vi "LaguerreGaussianBeam.vi"(0 "beam parameters":T1={"amplitudeMatrix"=[], "SLM width (m)"=0.01498, "SLM height (m)"=0.01092, "wavelength (m)"=6.33e-07, "Resolution x"=1920, "Resolution y"=1080} caption="Beam Parameters, dependant on SLM and LASER" {"Resolution x" format="%#.0f"; "SLM width (m)" format="%_6f"; "SLM height (m)" format="%#_6f"}, 1 "x centre":dbl, 2 "l":i16, 3 "p":i16 min=0 step=1, 4 "beam waist w0 (in m; default 1E-4 = 0.1mm)":dbl=0.0001 format="%.2p", 5 "Phase rotation":dbl min=-6.2832 max=6.28318530718 step=0.01570796326, 6 "y centre":dbl, 7 "Correction beam waist wc \n(in m; default 1 meter)":dbl=1.0 format="%.2p") -> (8 "Laguerre-Gaussian beam":T1={"amplitudeMatrix"=[], "SLM width (m)"=0.01498, "SLM height (m)"=0.01092, "wavelength (m)"=6.33e-07, "Resolution x"=1920, "Resolution y"=1080} caption="Beam Parameters, dependant on SLM and LASER" {"Resolution x" format="%#.0f"; "SLM width (m)" format="%_6f"; "SLM height (m)" format="%#_6f"})   [LabVIEW 2024]
uses:
  typeDefs/BPandSLM.ctl
panel:
  out "min value":dbl
  out "max value":dbl
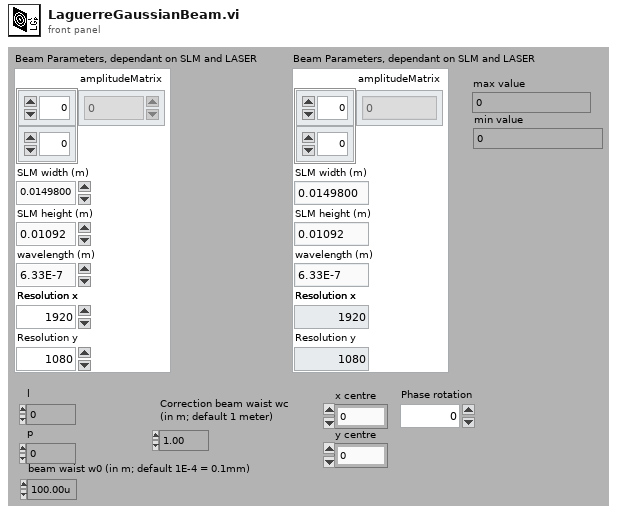
[diagram p1: front panel]
types:
  T1 = typedef "BPandSLM.ctl" = cluster{"amplitudeMatrix":csg[][], "SLM width (m)":dbl, "SLM height (m)":dbl, "wavelength (m)":dbl, "Resolution x":u32, "Resolution y":u32}
  T2 = cluster{"x values":dbl[], "laguerre polynomial values":dbl[]}
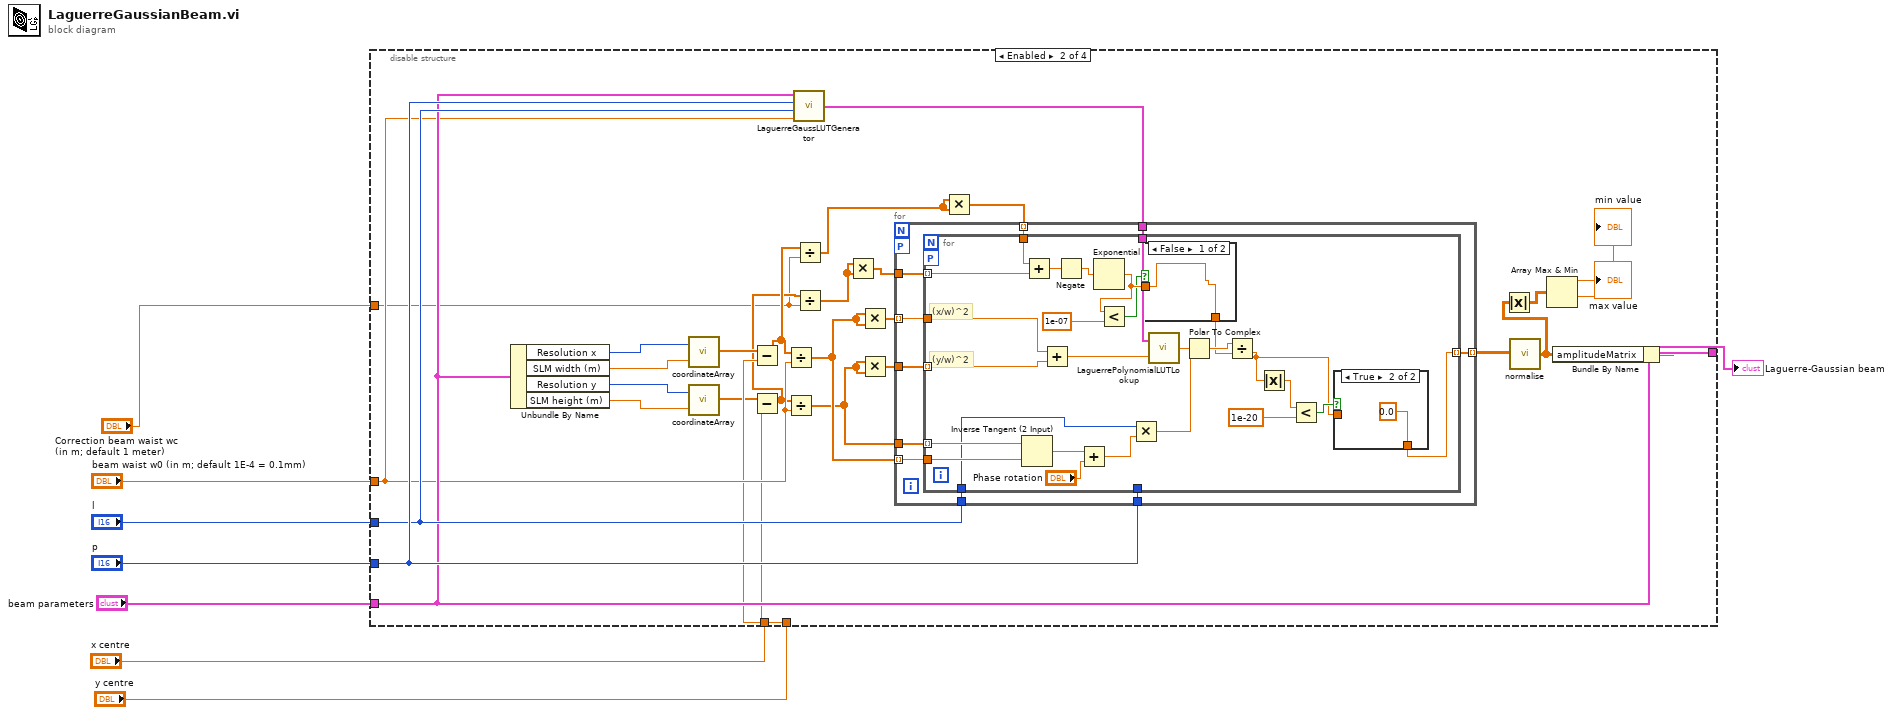
[diagram p0: block diagram]
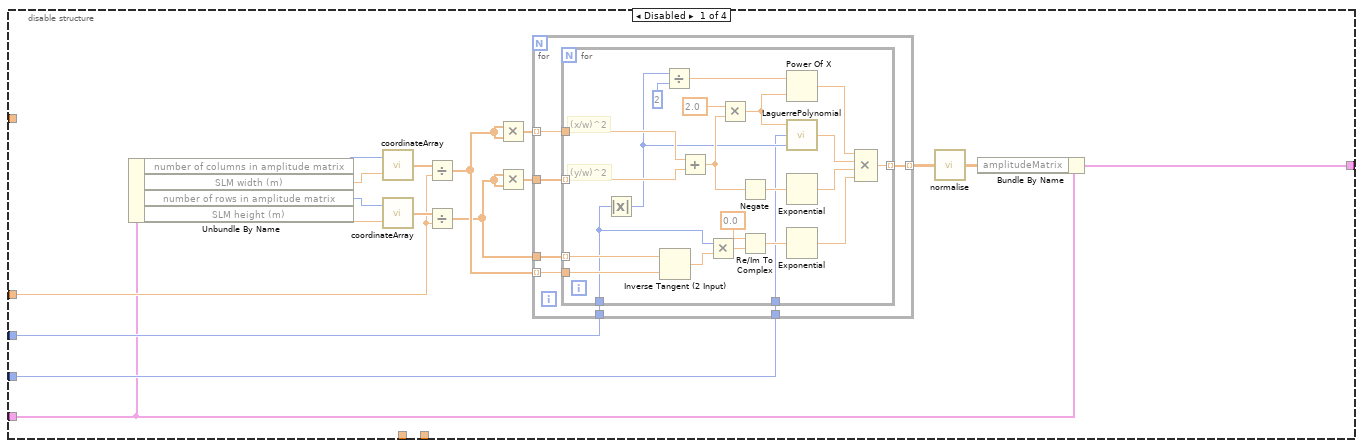
[diagram p2: hidden frame]
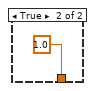
[diagram p4: hidden frame]
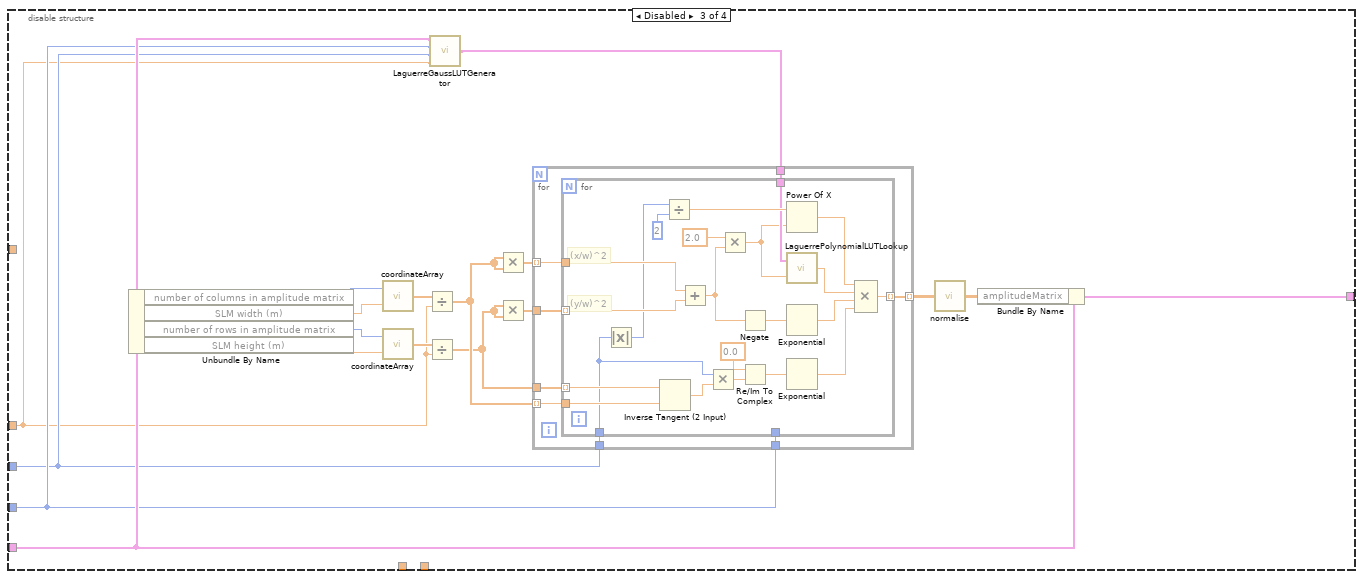
[diagram p5: hidden frame]
diagram:
  n1 = disable-structure shown="Enabled" {
    disable-tunnel: [w25 w84 w142 _] -> w2
    disable-tunnel: "p" -> [w12 w77 w127 _]
    disable-tunnel: "l" -> [w11 w76 w126 _]
    disable-tunnel: "beam waist w0 (in m; default 1E-4 = 0.1mm)" -> [w10 w74 w125 _]
    disable-tunnel: "beam parameters" -> [w9 w75 w128 _]
    disable-tunnel: "x centre" -> [_ w71 _ _]
    disable-tunnel: "y centre" -> [_ w72 _ _]
    disable-tunnel: "Correction beam waist wc \n(in m; default 1 meter)" -> [_ w64 _ _]
    frame Disabled {
      n2 = Unbundle By Name(w9) -> ("number of columns in amplitude matrix"=w24:i32, "SLM width (m)"=w14:dbl, "number of rows in amplitude matrix"=w23:i32, "SLM height (m)"=w13:dbl)
      n3 = call "coordinateArray.vi"("width of represented x (or y) range (in m; default 1E-3=1mm)"=w14, "array size (default 64)"=w24) -> ("x array"=w22:sgl[])
      n4 = call "coordinateArray.vi"("width of represented x (or y) range (in m; default 1E-3=1mm)"=w13, "array size (default 64)"=w23) -> ("x array"=w21:sgl[])
      n5 = Divide(x=w22, y=w10) -> (x/y=w18:dbl[])
      n6 = Divide(x=w21, y=w10) -> (x/y=w17:dbl[])
      n7 = Multiply(x=w18, y=w18) -> (x*y=w20:dbl[])
      n8 = Multiply(x=w17, y=w17) -> (x*y=w19:dbl[])
      n9 = for {
        tunnel: [w32] -> w16 mode=indexing
        tunnel: w20 -> [w31] mode=indexing
        tunnel: w19 -> [w30]
        tunnel: w18 -> [w29] mode=indexing
        tunnel: w17 -> [w28]
        tunnel: w11 -> [w27]
        tunnel: w12 -> [w26]
        n10 = for {
          tunnel: [w53] -> w32 mode=indexing
          tunnel: w31 -> [w52]
          tunnel: w30 -> [w51] mode=indexing
          tunnel: w29 -> [w41]
          tunnel: w28 -> [w40] mode=indexing
          tunnel: w27 -> [w37]
          tunnel: w26 -> [w33]
          # "(y/w)^2"
          # "(x/w)^2"
          n11 = Absolute Value(x=w37) -> (abs(x)=w34:i16)
          n12 = Inverse Tangent (2 Input)(1:w41, 2:w40) -> (0:w44:dbl)
          n13 = Divide(x=w34, y=i16 2) -> (x/y=w38:dbl)
          n14 = Add(x=w52, y=w51) -> (x+y=w48:dbl)
          n15 = Multiply(x=w37, y=w44) -> (x*y=w45:dbl)
          n16 = Multiply(x=2.0, y=w48) -> (x*y=w35:dbl)
          n17 = Negate(x=w48) -> (-x=w54:dbl)
          n18 = Re/Im To Complex(1:w45, 2:0.0 ("x")) -> (0:w46:cdb)
          n19 = Power Of X(1:w35, 2:w38) -> (0:w49:dbl)
          n20 = call "LaguerrePolynomial.vi"("a"=w34, "n"=w33, "x"=w35) -> ("associated Laguerre polynomial (n,a,x)"=w36:dbl)
          n21 = Exponential(1:w54) -> (0:w47:dbl)
          n22 = Exponential(1:w46) -> (0:w42:cdb)
          n23 = Compound Arithmetic op=MULTIPLY(w49, w36, w47, w42) -> (w53:cdb)
        }
      }
      n24 = call "normalise.vi"("amplitude matrix"=w16) -> ("normalised amplitude matrix"=w15:cdb[][])
      n25 = Bundle By Name(cluster=w9, "amplitudeMatrix"=w15) -> (w25:T1)
    }
    frame Enabled {
      n26 = Unbundle By Name(w75) -> ("Resolution x"=w83:u32, "SLM width (m)"=w79:dbl, "Resolution y"=w82:u32, "SLM height (m)"=w78:dbl)
      n27 = call "coordinateArray.vi"("width of represented x (or y) range (in m; default 1E-3=1mm)"=w79, "array size (default 64)"=w83) -> ("x array"=w70:sgl[])
      n28 = call "coordinateArray.vi"("width of represented x (or y) range (in m; default 1E-3=1mm)"=w78, "array size (default 64)"=w82) -> ("x array"=w67:sgl[])
      n29 = Subtract(x=w70, y=w71) -> (x-y=w66:dbl[])
      n30 = Subtract(x=w67, y=w72) -> (x-y=w65:dbl[])
      n31 = Divide(x=w66, y=w74) -> (x/y=w69:dbl[])
      n32 = Divide(x=w65, y=w74) -> (x/y=w68:dbl[])
      n33 = call "LaguerreGaussLUTGenerator.vi"("beam waist w0 (in m; default 1E-4 = 0.1mm)"=w74, "l"=w76, "p"=w77, "beam parameters"=w75) -> ("Look-up Table"=w73:T2)
      n34 = Divide(x=w66, y=w64) -> (x/y=w62:dbl[])
      n35 = Divide(x=w65, y=w64) -> (x/y=w63:dbl[])
      n36 = Multiply(x=w63, y=w63) -> (x*y=w60:dbl[])
      n37 = Multiply(x=w69, y=w69) -> (x*y=w81:dbl[])
      n38 = Multiply(x=w68, y=w68) -> (x*y=w80:dbl[])
      n39 = Multiply(x=w62, y=w62) -> (x*y=w61:dbl[])
      n40 = for {
        tunnel: [w94] -> w55 mode=indexing
        tunnel: w81 -> [w93] mode=indexing
        tunnel: w80 -> [w92]
        tunnel: w69 -> [w91] mode=indexing
        tunnel: w68 -> [w90]
        tunnel: w76 -> [w89]
        tunnel: w77 -> [w88]
        tunnel: w73 -> [w87]
        workers-P: _ -> [_]
        tunnel: w60 -> [w86]
        tunnel: w61 -> [w85] mode=indexing
        n41 = for {
          tunnel: [w99] -> w94 mode=indexing
          tunnel: w93 -> [w120]
          tunnel: w92 -> [w119] mode=indexing
          tunnel: w91 -> [w118]
          tunnel: w90 -> [w117] mode=indexing
          tunnel: w89 -> [w116]
          tunnel: w88 -> [_]
          tunnel: w87 -> [w115]
          workers-P: _ -> [_]
          tunnel: w86 -> [w112] mode=indexing
          tunnel: w85 -> [w111]
          # "(y/w)^2"
          # "(x/w)^2"
          n42 = Inverse Tangent (2 Input)(1:w118, 2:w117) -> (0:w96:dbl)
          n43 = Add(x=w111, y=w112) -> (x+y=w109:dbl)
          n44 = Add(x=w120, y=w119) -> (x+y=w110:dbl)
          n45 = Negate(x=w109) -> (-x=w108:dbl)
          n46 = Add(x=w96, y="Phase rotation") -> (x+y=w97:dbl)
          n47 = Exponential(1:w108) -> (0:w106:dbl)
          n48 = Less?(x=w106, y=1e-07) -> (x < y?=w103:bool)
          n49 = Multiply(x=w116, y=w97) -> (x*y=w114:dbl)
          n50 = case shown="False" w103 {
            tunnel: w106 -> [w123 _]
            tunnel: [w123 1.0 ("y")] -> w104
            frame False {
            }
            frame True {
            }
          }
          n51 = call "LaguerrePolynomialLUTLookup.vi"("x"=w110, "Look-up Table"=w115) -> ("Function value"=w113:dbl)
          n52 = Polar To Complex(1:w114, 2:w113) -> (0:w105:cdb)
          n53 = Divide(x=w105, y=w104) -> (x/y=w98:cdb)
          n54 = Absolute Value(x=w98) -> (abs(x)=w102:dbl)
          n55 = Less?(x=w102, y=1e-20) -> (x < y?=w100:bool)
          n56 = case shown="True" w100 {
            tunnel: w98 -> [w121 _]
            tunnel: [w121 0.0 ("y")] -> w99
            frame False {
            }
            frame True {
            }
          }
        }
      }
      n57 = call "normalise.vi"("amplitude matrix"=w55) -> ("normalised amplitude matrix"=w56:cdb[][])
      n58 = Absolute Value(x=w56) -> (abs(x)=w59:dbl[][])
      n59 = Array Max & Min(array=w59) -> (max value=→"max value":dbl, min value=→"min value":dbl)  [unwired: 2 out]
      n60 = Bundle By Name(cluster=w75, "amplitudeMatrix"=w56) -> (w84:T1)
    }
    frame Disabled {
      n61 = Unbundle By Name(w128) -> ("number of columns in amplitude matrix"=w141:i32, "SLM width (m)"=w131:dbl, "number of rows in amplitude matrix"=w140:i32, "SLM height (m)"=w130:dbl)
      n62 = call "coordinateArray.vi"("width of represented x (or y) range (in m; default 1E-3=1mm)"=w131, "array size (default 64)"=w141) -> ("x array"=w139:sgl[])
      n63 = call "coordinateArray.vi"("width of represented x (or y) range (in m; default 1E-3=1mm)"=w130, "array size (default 64)"=w140) -> ("x array"=w138:sgl[])
      n64 = Divide(x=w139, y=w125) -> (x/y=w135:dbl[])
      n65 = Divide(x=w138, y=w125) -> (x/y=w134:dbl[])
      n66 = call "LaguerreGaussLUTGenerator.vi"("beam waist w0 (in m; default 1E-4 = 0.1mm)"=w125, "l"=w126, "p"=w127, "beam parameters"=w128) -> ("Look-up Table"=w129:T2)
      n67 = Multiply(x=w135, y=w135) -> (x*y=w137:dbl[])
      n68 = Multiply(x=w134, y=w134) -> (x*y=w136:dbl[])
      n69 = for {
        tunnel: [w150] -> w133 mode=indexing
        tunnel: w137 -> [w149] mode=indexing
        tunnel: w136 -> [w148]
        tunnel: w135 -> [w147] mode=indexing
        tunnel: w134 -> [w146]
        tunnel: w126 -> [w145]
        tunnel: w127 -> [w144]
        tunnel: w129 -> [w143]
        n70 = for {
          tunnel: [w171] -> w150 mode=indexing
          tunnel: w149 -> [w170]
          tunnel: w148 -> [w169] mode=indexing
          tunnel: w147 -> [w159]
          tunnel: w146 -> [w158] mode=indexing
          tunnel: w145 -> [w155]
          tunnel: w144 -> [_]
          tunnel: w143 -> [w153]
          # "(y/w)^2"
          # "(x/w)^2"
          n71 = Absolute Value(x=w155) -> (abs(x)=w154:i16)
          n72 = Inverse Tangent (2 Input)(1:w159, 2:w158) -> (0:w162:dbl)
          n73 = Divide(x=w154, y=i16 2) -> (x/y=w156:dbl)
          n74 = Add(x=w170, y=w169) -> (x+y=w166:dbl)
          n75 = Multiply(x=w155, y=w162) -> (x*y=w163:dbl)
          n76 = Multiply(x=2.0, y=w166) -> (x*y=w152:dbl)
          n77 = Negate(x=w166) -> (-x=w172:dbl)
          n78 = Re/Im To Complex(1:w163, 2:0.0 ("x")) -> (0:w164:cdb)
          n79 = Power Of X(1:w152, 2:w156) -> (0:w167:dbl)
          n80 = call "LaguerrePolynomialLUTLookup.vi"("x"=w152, "Look-up Table"=w153) -> ("Function value"=w151:dbl)
          n81 = Exponential(1:w172) -> (0:w165:dbl)
          n82 = Exponential(1:w164) -> (0:w160:cdb)
          n83 = Compound Arithmetic op=MULTIPLY(w167, w151, w165, w160) -> (w171:cdb)
        }
      }
      n84 = call "normalise.vi"("amplitude matrix"=w133) -> ("normalised amplitude matrix"=w132:cdb[][])
      n85 = Bundle By Name(cluster=w128, "amplitudeMatrix"=w132) -> (w142:T1)
    }
    frame Disabled {
    }
  }
  "Laguerre-Gaussian beam" <- w2
